vi "distance_to_segment_along_heading.vi"(8 "Heading (deg)":dbl, 9 "Segment Point 2":T1 {"North" format="%#_10f"; "East" format="%#_8f"}, 10 "Segment Point 1":T1 {"North" format="%#_10f"; "East" format="%#_8f"}, 11 "Boat Point":T1 {"North" format="%#_10f"; "East" format="%#_8f"}) -> ()   [LabVIEW 2013]
uses:
  Data/TypeDefs/UTM Location.ctl
panel:
  out "Distance from boat to intersection point":dbl
  out "Intersection point":T1 {"North" format="%#_10f"; "East" format="%#_8f"}
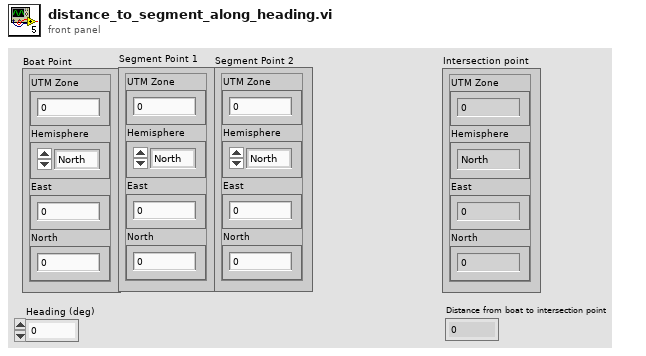
[diagram p1: front panel]
types:
  T1 = typedef "UTM Location.ctl" = cluster{"UTM Zone":dbl, "Hemisphere":enum16{"North", "South"}, "East":dbl, "North":dbl}
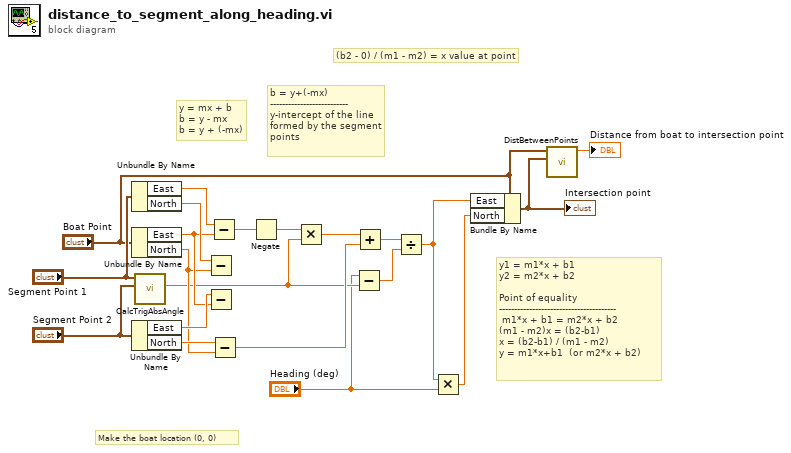
[diagram p0: block diagram]
diagram:
  # "y = mx + b\nb = y - mx\nb = y + (-mx)"
  # "(b2 - 0) / (m1 - m2) = x value at point"
  # "b = y+(-mx)\n--------------------------\ny-intercept of the line formed by the segment points"
  # "Make the boat location (0, 0)"
  # "y1 = m1*x + b1\ny2 = m2*x + b2\n\nPoint of equality\n---------------------------------------\n m1*x + b1 = m2*x + b2\n(m1 - m2)x = (b2-b1)\nx = (b2-b1) / (m1 - m2)\ny = m1*x+b1  (or m2*x + b2)"
  n1 = Unbundle By Name("Segment Point 1") -> ("East"=w19:dbl, "North"=w17:dbl)
  n2 = Unbundle By Name("Boat Point") -> ("East"=w16:dbl, "North"=w14:dbl)
  n3 = Unbundle By Name("Segment Point 2") -> ("East"=w18:dbl, "North"=w15:dbl)
  n4 = call "CalcTrigAbsAngle.vi"("Point 2"="Segment Point 2", "Point 1"="Segment Point 1") -> ("Angle between points (deg)"=w8:dbl)  [unwired: 8 in, 1 out]
  n5 = Subtract(x=w17, y=w14) -> ()  [unwired: 1 out]
  n6 = Subtract(x=w18, y=w16) -> ()  [unwired: 1 out]
  n7 = Subtract(x=w19, y=w16) -> (x-y=w13:dbl)
  n8 = Subtract(x=w15, y=w14) -> (x-y=w10:dbl)
  n9 = Negate(x=w13) -> (-x=w12:dbl)
  n10 = Multiply(x=w12, y=w8) -> (x*y=w11:dbl)
  n11 = Subtract(x="Heading (deg)", y=w8) -> (x-y=w7:dbl)
  n12 = Add(x=w11, y=w10) -> (x+y=w9:dbl)
  n13 = Divide(x=w9, y=w7) -> (x/y=w6:dbl)
  n14 = Multiply(x=w6, y="Heading (deg)") -> (x*y=w4:dbl)
  n15 = Bundle By Name(cluster="Boat Point", "East"=w6, "North"=w4) -> (w2:T1)
  "Intersection point" <- w2
  n16 = call "DistBetweenPoints.vi"("UTM Location 2"=w2, "UTM Location 1"="Boat Point") -> ("Distance from 1 to 2"=→"Distance from boat to intersection point":dbl)  [unwired: 9 in]
